vi "SMTP Email Convert Attach to UTF8.vi"(2 "error in":errorcluster, 3 "attachments":T1(array[cluster])) -> (0 "error out":errorcluster, 1 "UTF-8 Attachments":T1(array[cluster]))   [LabVIEW 2011, in "NewNI_SMTPEmail.lvlib"]
uses:
  NewNI_SMTPEmail.lvlib
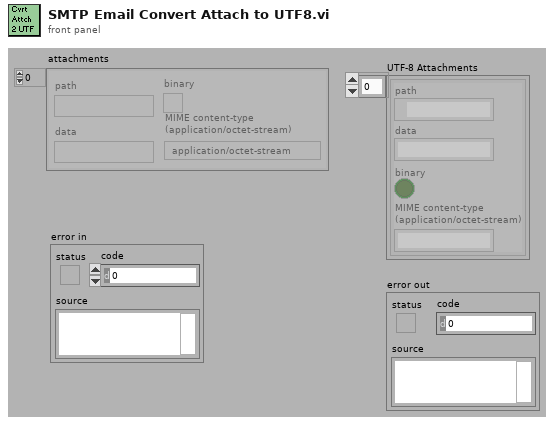
[diagram p1: front panel]
types:
  T1 = cluster{"path":path, "data":string, "binary":bool, "MIME content-type \n(application/octet-stream)":string}[]
  T2 = cluster{"path":path, "data":string, "binary":bool, "MIME content-type \n(application/octet-stream)":string}
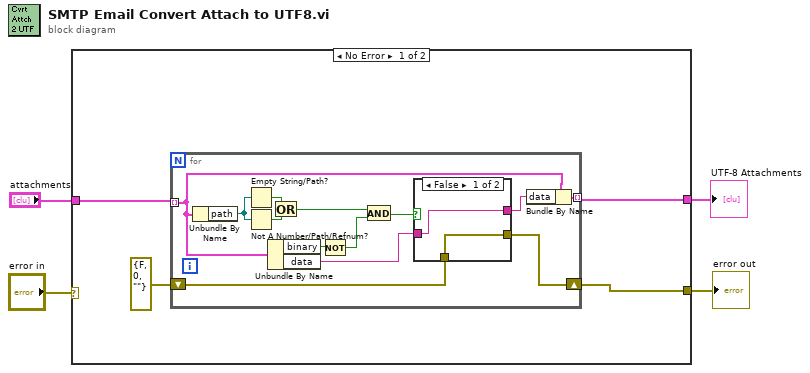
[diagram p0: block diagram]
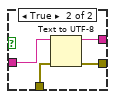
[diagram p2: hidden frame]
diagram:
  n1 = case shown="No Error" "error in" {
    selector: "error in" -> [_ w29]
    tunnel: [w8 w28] -> w4
    tunnel: [w7 w29] -> w3
    tunnel: "attachments" -> [w5 w28]
    frame No Error {
      n2 = for {
        tunnel: w5 -> [w11] mode=indexing
        shift-right: [w13] -> w7
        shift-left: errorcluster {"status"=FALSE, "code"=0, "source"=""} ("error out") -> [w12]
        tunnel: [w9] -> w8 mode=indexing
        n3 = Unbundle By Name(w11) -> ("path"=w21:path)
        n4 = Empty String/Path?(string/path=w21) -> (empty?=w19:bool)
        n5 = Not A Number/Path/Refnum?(number/path/refnum=w21) -> (NaN/Path/Refnum?=w20:bool)
        n6 = Unbundle By Name(w11) -> ("binary"=w18:bool, "data"=w14:string)
        n7 = Or(x=w19, y=w20) -> (x .or. y?=w16:bool)
        n8 = Not(x=w18) -> (.not. x?=w17:bool)
        n9 = And(x=w16, y=w17) -> (x .and. y?=w15:bool)
        n10 = case shown="False" w15 {
          tunnel: w14 -> [w23 w27]
          tunnel: [w23 w26] -> w10
          tunnel: [w22 w25] -> w13
          tunnel: w12 -> [w22 w24]
          frame False {
          }
          frame True {
            n11 = Text to UTF-8(8:w24, 11:w27) -> (0:w25:errorcluster, 3:w26:string)
          }
        }
        n12 = Bundle By Name(cluster=w11, "data"=w10) -> (w9:T2)
      }
    }
    frame Error {
    }
  }
  "UTF-8 Attachments" <- w4
  "error out" <- w3
